vi "SaveHospInfo.vi"() -> (0 "Cancel?":bool=TRUE, 1 "Department 2":string, 2 "Hospital Address 2":string, 3 "Hospital Name 2":string)   [LabVIEW 2013, in "main.lvlib"]
uses:
  main.lvlib
  Controls/Enum Save Action Events.ctl
  Controls/SaveDataCluster.ctl
panel:
  in  "Department":string caption="Afdeling"
  in  "HospCancelBtn":bool
  in  "HospSaveBtn":bool
  in  "Address":string caption="Adresse"
  in  "Hospital":string
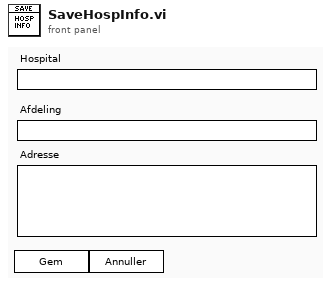
[diagram p1: front panel]
types:
  T1 = typedef "main.lvlib/SaveDataCluster.ctl" = cluster{"HospInfo":cluster{"Name":string, "Address":string, "Department":string}, "Pressure":cluster{"Pressure":dbl}, "DataPath":cluster{"DataPath":path}, "ReportPath":cluster{"Path":path, "Name":string}, "DICOM Info WL":cluster{"port":i32, "AEtitle":string, "host":string, "remoteAE":string}, "DICOM Info PACS":cluster{"port":i32, "AEtitle":string, "host":string, "remoteAE":string}, "ArmCalcMethod":dbl, "itemTags":string[], "DicomEncoding":u16, "JournalType":u16, "General Settings":cluster{"Hyphenation":bool, "Language":u16, "CellStr1":string, "CellStr2":string}, "Dicom Tags":string[][], "BT Serial":cluster{"Serial Number":string, "Side":string, "Ignore?":bool}[], "BT License":cluster{"License":string, "Accepted Serials":string[]}}
  T2 = typedef "main.lvlib/Enum Save Action Events.ctl" = enum16{"LoadReportPath", "SaveReportPath", "Load Graph Path", "Save Graph Path", "LoadDataPath", "SaveDataPath", "Load Template Path", "Save Template Path", "Load PressureFactor", "Save PressureFactor", "Init", "Load Listbox", "Save Listbox", "LoadHospInfo", "SaveHospInfo", "Load DICOM Activation", "Save DICOM Activation", "LoadDICOMInfoWL", "SaveDICOMInfoWL", "LoadDICOMInfoPACS", "SaveDICOMInfoPACS", "Load ArmCalcMethod", "Save ArmCalcMethod", "LoadItemTags", "SaveItemTags", "LoadDICOMEncoding", "SaveDICOMEncoding", "LoadJournalType", "SaveJournalType", "LoadAcqFilterType", "SaveAcqFilterType", "Load Sequence", "Save Sequence", "Load Acquisition Mode", "Save Acquisition Mode", "Load General Settings", "Save General Settings", "Load Language", "Save Language", "Load Dicom Tags", "Save Dicom Tags", "Load BT Serial", "Save BT Serial", "Load BT License", "Save BT License"}
  T3 = cluster{"Name":string, "Address":string, "Department":string}
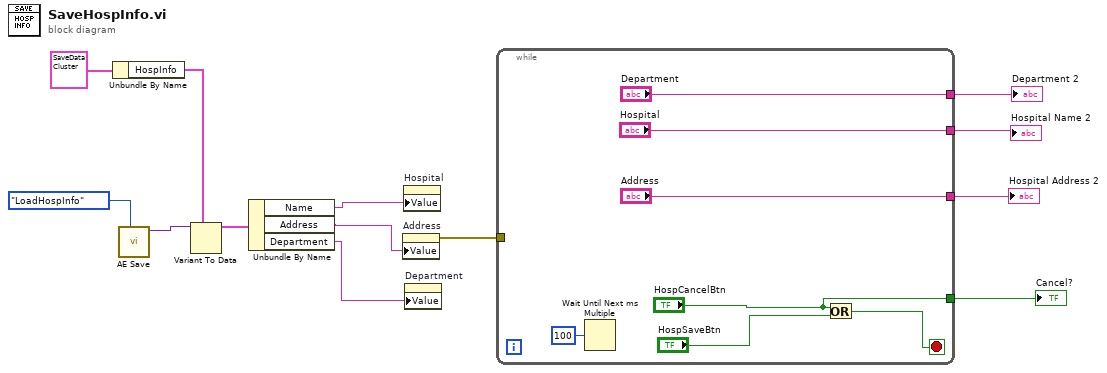
[diagram p0: block diagram]
diagram:
  n1 = Unbundle By Name(T1 {"HospInfo"={"Name"="", "Address"="", "Department"=""}, "Pressure"={"Pressure"=0.0}, "DataPath"={"DataPath"=path ""}, "ReportPath"={"Path"=path "", "Name"=""}, "DICOM Info WL"={"port"=0, "AEtitle"="", "host"="", "remoteAE"=""}, "DICOM Info PACS"={"port"=0, "AEtitle"="", "host"="", "remoteAE"=""}, "ArmCalcMethod"=0.0, "itemTags"=[], "DicomEncoding"=0, "JournalType"=0, "General Settings"={"Hyphenation"=FALSE, "Language"=0, "CellStr1"="", "CellStr2"=""}, "Dicom Tags"=[], "BT Serial"=[], "BT License"={"License"="", "Accepted Serials"=[]}} ("Data")) -> ("HospInfo"=w5:T3)
  n2 = call "AE Save.vi"("Action"=Enum_Save_Action_Events."LoadHospInfo") -> ("Anything"=w9:variant)  [unwired: 8 in, 1 out]
  n3 = Variant To Data(type=w5, Variant=w9) -> (data=w4:T3)  [unwired: 1 in, 1 out]
  n4 = Unbundle By Name(w4) -> ("Name"=w3:string, "Address"=w2:string, "Department"=w1:string)
  n5 = property on="Address" class="Str"("Value"=w2) -> (error out=w7:errorcluster)  [unwired: 2 in, 1 out]
  n6 = property on="Hospital" class="Str"("Value"=w3) -> ()  [unwired: 2 in, 2 out]
  n7 = property on="Department" class="Str"("Value"=w1) -> ()  [unwired: 2 in, 2 out]
  n8 = while {
    tunnel: ["Address"] -> w13
    tunnel: ["Hospital"] -> w12
    tunnel: ["HospCancelBtn"] -> w11
    tunnel: ["Department"] -> w10
    tunnel: w7 -> [_]
    stop <- w15 stop-if-true
    n9 = Wait Until Next ms Multiple(millisecond multiple=u32 100) -> ()  [unwired: 1 out]
    n10 = Or(x="HospCancelBtn", y="HospSaveBtn") -> (x .or. y?=w15:bool)
  }
  "Hospital Name 2" <- w12
  "Hospital Address 2" <- w13
  "Cancel?" <- w11
  "Department 2" <- w10
